vi "画对角线.vi"(10 "Caliper Results (两条直线对角线)":sgl[][](array[numeric]), 11 "引用句柄输入":T1) -> ()   [LabVIEW 2014]
uses:
  <vilib>/vision/Image Controls.llb/IMAQ Image.ctl
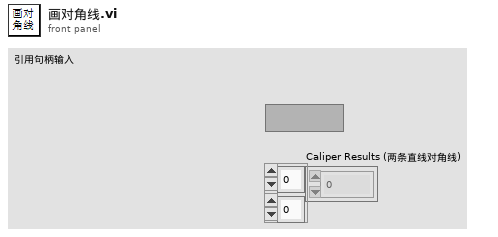
[diagram p1: front panel]
types:
  T1 = typedef "IMAQ Image.ctl" = refnum<image>
  T2 = cluster{"output string":sgl, "output string":sgl}
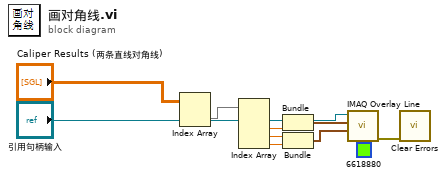
[diagram p0: block diagram]
diagram:
  n1 = Index Array(array="Caliper Results (两条直线对角线)") -> (element=w2:sgl[])  [unwired: 2 in]
  n2 = Index Array(array=w2) -> (element #1=w3:sgl, element #2=w4:sgl, element #3=w5:sgl, element #4=w6:sgl)  [unwired: 4 in]
  n3 = Bundle("output string"=w3, "output string"=w4) -> (w7:T2)  [unwired: 1 in]
  n4 = Bundle("output string"=w5, "output string"=w6) -> (w11:T2)  [unwired: 1 in]
  n5 = call "IMAQ Overlay Line"("Color"=u32 6618880, "End Point"=w11, "Start Point"=w7, "Image"="引用句柄输入") -> ("error out"=w8:errorcluster)  [unwired: 6 in, 1 out]
  n6 = call <vilib>:"Clear Errors.vi"("error in (no error)"=w8) -> ()  [unwired: 5 in, 2 out]
